vi "writeRejectCmdEvnt.vi"(8 "error in (no error)":errorcluster, 10 "RejectedCommand":refnum<user-event>, 11 "ElectrometerController in":refnum<class "ElectrometerController.lvclass">) -> (0 "error out":errorcluster, 3 "ElectrometerController out":refnum<class "ElectrometerController.lvclass">)   [LabVIEW 2016, in "ElectrometerController.lvclass"]
uses:
  ElectrometerController.lvclass
  ts_electrometeruserevents/Typedefs/RejectedCommand.ctl
  ts_electrometeruserevents/Typedefs/CommandValue.ctl
  ts_electrometeruserevents/Typedefs/StateValue.ctl
  ElectrometerController.lvclass/ElectrometerController.ctl
  ts_electrometeruserevents/Typedefs/ElectrometerTypedefs.lvlib
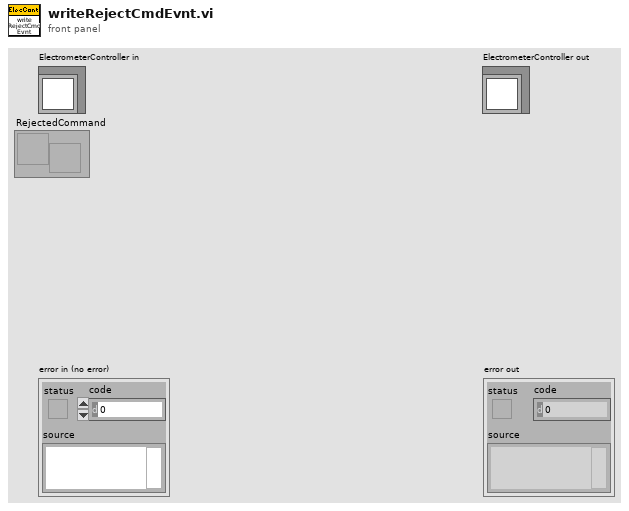
[diagram p1: front panel]
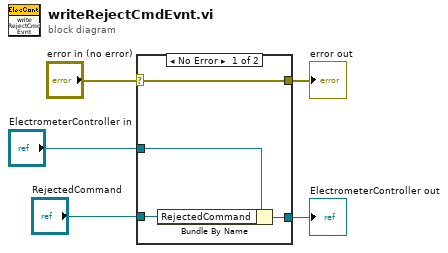
[diagram p0: block diagram]
diagram:
  n1 = case shown="No Error" "error in (no error)" {
    selector: "error in (no error)" -> [w6 w11]
    tunnel: [w6 w11] -> w4
    tunnel: [w8 w10] -> w2
    tunnel: "ElectrometerController in" -> [w9 w10]
    tunnel: "RejectedCommand" -> [w7 _]
    frame No Error {
      n2 = Bundle By Name(cluster=w9, "RejectedCommand"=w7) -> (w8:refnum<class "ElectrometerController.lvclass">)
    }
    frame Error {
    }
  }
  "error out" <- w4
  "ElectrometerController out" <- w2
